vi "RFmx LUT Configuration.vi"(7 "Selector String":string, 8 "error in (no error)":errorcluster, 10 "RFmxLUT Configuration":T1={"Threshold Enabled"=1, "Threshold Type"=0, "Threshold Level (dB or dBm)"=-20.0, "LUT Step Size (dB)"=0.1, "LUT Correction Type"=0, " LUT Type"=0} {"LUT Type" items=["Log", "Linear"]; "LUT Correction Type" items=["Magnitude and Phase", "Magnitude Only", "Phase Only"]; "Threshold Level (dB or dBm)" format="%.2g"; "Threshold Type" items=["Relative", "Absolute"]; "Threshold Enabled" items=["False", "True"]}, 11 "Instrument Handle In":refnum<k21>) -> (0 "error out":errorcluster, 3 "Instrument Handle Out":refnum<k21>)   [LabVIEW 2016, in "DPD.lvlib"]
uses:
  DPD.lvlib
  Typedefs/RFmx LUT Configuration.ctl
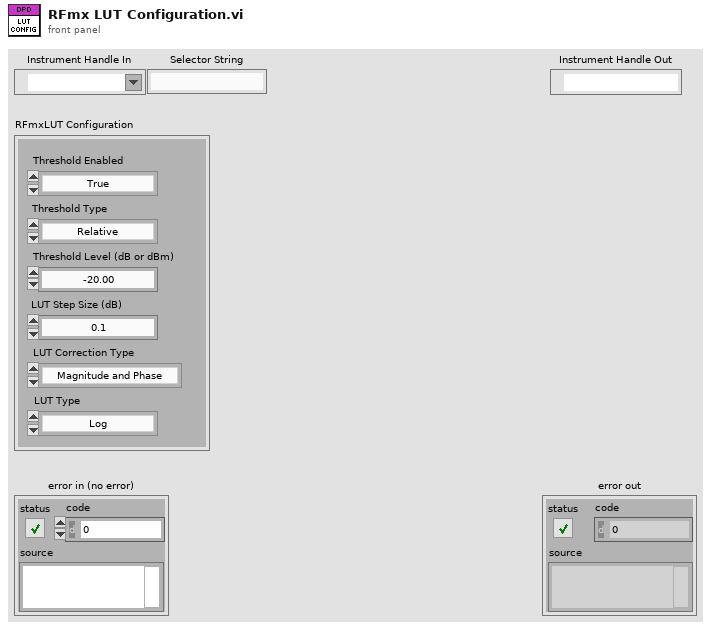
[diagram p1: front panel]
types:
  T1 = typedef "DPD.lvlib/RFmx LUT Configuration.ctl" = cluster{"Threshold Enabled":i32, "Threshold Type":i32, "Threshold Level (dB or dBm)":dbl, "LUT Step Size (dB)":dbl, "LUT Correction Type":i32, " LUT Type":i32}
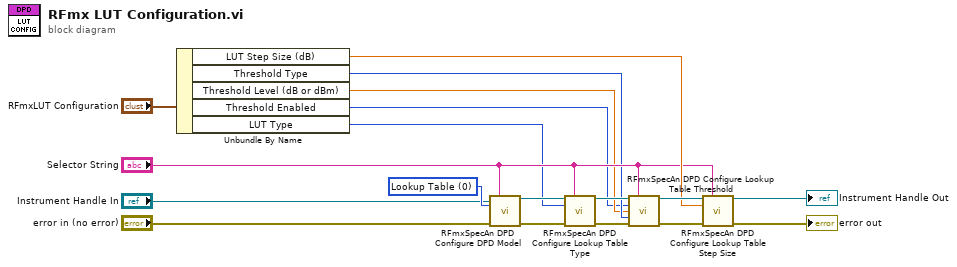
[diagram p0: block diagram]
diagram:
  w18 = 0 items=["Lookup Table", "Memory Polynomial", "Generalized Memory Polynomial"] ("DPD Model")
  n1 = Unbundle By Name("RFmxLUT Configuration") -> ("LUT Step Size (dB)"=w8:dbl, "Threshold Type"=w6:i32, "Threshold Level (dB or dBm)"=w5:dbl, "Threshold Enabled"=w4:i32, "LUT Type"=w3:i32)
  n2 = call <vilib>:"RFmxSpecAn DPD Configure DPD Model.vi"("Instrument Handle In"="Instrument Handle In", "Selector String"="Selector String", "DPD Model"=w18, "error in (no error)"="error in (no error)") -> ("Instrument Handle Out"=w13:refnum<k21>, "error out"=w12:errorcluster)  [unwired: 10 in]
  n3 = call <vilib>:"RFmxSpecAn DPD Configure Lookup Table Type.vi"("Instrument Handle In"=w13, "Selector String"="Selector String", "DPD LUT Type"=w3, "error in (no error)"=w12) -> ("Instrument Handle Out"=w11:refnum<k21>, "error out"=w10:errorcluster)  [unwired: 10 in]
  n4 = call <vilib>:"RFmxSpecAn DPD Configure Lookup Table Threshold.vi"("Instrument Handle In"=w11, "Selector String"="Selector String", "Threshold Enabled"=w4, "Threshold Level (dB or dBm)"=w5, "Threshold Type"=w6, "error in (no error)"=w10) -> ("Instrument Handle Out"=w17:refnum<k21>, "error out"=w16:errorcluster)  [unwired: 8 in]
  n5 = call <vilib>:"RFmxSpecAn DPD Configure Lookup Table Step Size.vi"("Instrument Handle In"=w17, "Selector String"="Selector String", "Step Size (dB)"=w8, "error in (no error)"=w16) -> ("Instrument Handle Out"=→"Instrument Handle Out":refnum<k21>, "error out"=→"error out":errorcluster)  [unwired: 10 in]
